vi "SetUpMotor.vi"(8 "Error In":errorcluster, 10 "Serial Number":string="27004535", 11 "LabJack in":refnum<k24>) -> (0 "Error Out":errorcluster, 3 "reference out":refnum<k24>)   [LabVIEW 2018, in "ThorlabsLabJack.lvlib" / "ThorlabsLabJack.lvclass"]
uses:
  ThorlabsLabJack.lvclass
  C:/AME Test Engineering/LabVIEW/PPLs/Axis/Thorlabs/Thorlabs.MotionControl.IntegratedStepperMotorsCLI.dll
  PPLs/Axis/Thorlabs/Thorlabs.MotionControl.IntegratedStepperMotorsCLI.dll
  C:/AME Test Engineering/LabVIEW/PPLs/Axis/DLLs/Thorlabs.MotionControl.GenericMotorCLI.dll
  PPLs/Axis/DLLs/Thorlabs.MotionControl.GenericMotorCLI.dll
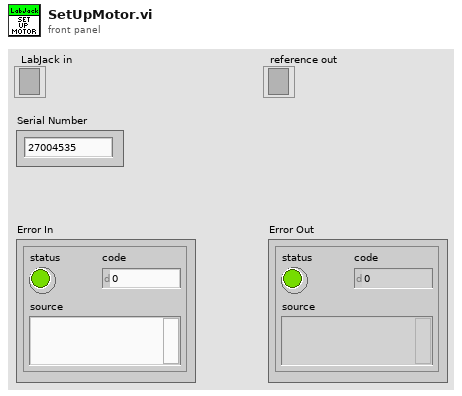
[diagram p1: front panel]
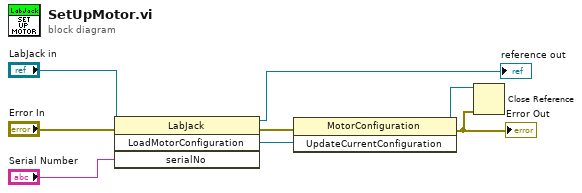
[diagram p0: block diagram]
diagram:
  n1 = invoke class="LabJack" method="LoadMotorConfiguration"(reference="LabJack in", error in="Error In", "serialNo"="Serial Number") -> (reference out=→"reference out":refnum<k24>, error out=w6:errorcluster, "LoadMotorConfiguration"=w5:refnum<k24>)  [unwired: 1 in, 1 out]
  n2 = invoke class="MotorConfiguration" method="UpdateCurrentConfiguration"(reference=w5, error in=w6) -> (reference out=w1:refnum<k24>, error out=w2:errorcluster)  [unwired: 1 in, 1 out]
  "Error Out" <- w2
  n3 = Close Reference(reference=w1, error in (no error)=w2) -> ()  [unwired: 1 out]
